vi "Set Ziro.vi"(6 "Direction":T1, 7 "init":bool, 8 "error in (no error)":errorcluster, 11 "Stand in":refnum<class "Stand.lvclass">) -> (0 "error out":errorcluster, 3 "Stand out":refnum<class "Stand.lvclass">)   [LabVIEW 2019, in "Stand.lvclass"]
uses:
  Stand.lvclass
  TypeDef/Direction.ctl
  D:/GIT H4000/H4000/src/Device_class/Device.lvclass
  Stand.lvclass/Stand.ctl
  Valve Mode.ctl
  Device_class/Device.lvclass/Device.ctl
  NeedleValve_class/Cmd.ctl
  ee99d7a0-1d06-4dde-a5e8-abf916667462.vi
  f8234472-8bf1-448c-8c25-8d9f60be58e1.vi
  6b2010b2-6e4b-4e14-9c16-a142e06b5f9e.vi
  Valve State Mode.vi
  Valve State Mode.vi/810e184e-eeb6-4027-a8ae-1422f3ce3d45.vi
  Valve State Mode.vi/57bd4a65-f3dc-44f5-8d68-677c2a197570.vi
  Valve State Mode.vi/03b2f9e4-fceb-4725-9b90-3fd10082a088.vi
  Valve State Mode.vi/2785bab5-dd59-4d13-b638-b9157202fa4a.vi
  Valve State Mode.vi/50faa4b8-a9b4-4cc6-ab66-55c42b424fcd.vi
  Valve State Mode.vi/c882c3fe-b7a7-4419-8f9b-6788aa23338b.vi
  Valve State Mode.vi/3d0d09bd-48e8-482f-b1e2-a36b2bb65234.vi
  Valve State Mode.vi/33d3f26a-dc4a-4f56-bf0a-61d04c5d7434.vi
  Valve State Mode.vi/52af9d47-24d1-4057-80bf-8d93bfb3d17d.vi
  Valve State Mode.vi/bbc9916c-129f-4456-975e-9c3ae3d5db66.vi
  Valve State Mode.vi/a6106d78-2bf9-477e-b655-d47fad07ddfe.vi
  Valve State Mode.vi/e2916439-03c6-4471-bb40-42242a636e27.vi
  Valve State Mode.vi/094228cb-a119-423c-9af8-5a16f059a318.vi
  Valve State Mode.vi/bf5ad1e6-a0ae-4579-ad74-ca8f304cb7cf.vi
  Valve State Mode.vi/eb4d2b76-f0f0-4e1d-bda0-609c5f37b4e7.vi
  Const All Valve.vi
  FPGA/TypeDef/DO index.ctl
  FPGA_API_class/FPGA API.lvclass
  Device_class/Device.lvclass
  NeedleValve_class/NeedleValve.lvclass
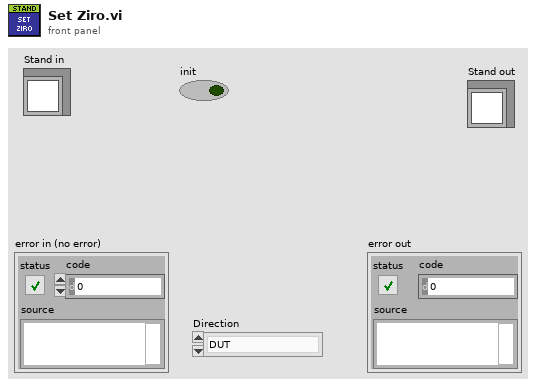
[diagram p1: front panel]
types:
  T1 = typedef "Direction.ctl" = enum8{"DUT", "Chamber"}
  T2 = typedef "DO index.ctl" = u8
  T3 = typedef "SP_TYPE.ctl" = enum16{"ERROR", "ZIRO", "BASE", "SP"}
  T4 = typedef "Valve Mode.ctl" = enum16{"Filling DUT", "Filling Chamber", "Pump Pressure DUT", "Pump Pressure Chamber", "Haskel Pressure DUT", "Haskel Pressure Chamber", "Slow Release DUT", "Slow Release Chamber", "Fast Release DUT", "Fast Release Chamber", "Fast Release DUT and Chamber", "Leak Pressure DUT", "Leak Pressure Chamber", "Back Pressure DUT", "Back Pressure Chamber", "Fully Closed", "Drain", "Block DUT", "Block Chamber", "filling dut down", "filling chamber down"}
  T5 = typedef "NeedleValve.lvclass/Cmd.ctl" = enum16{"Open", "Close", "Stop", "Prep open"}
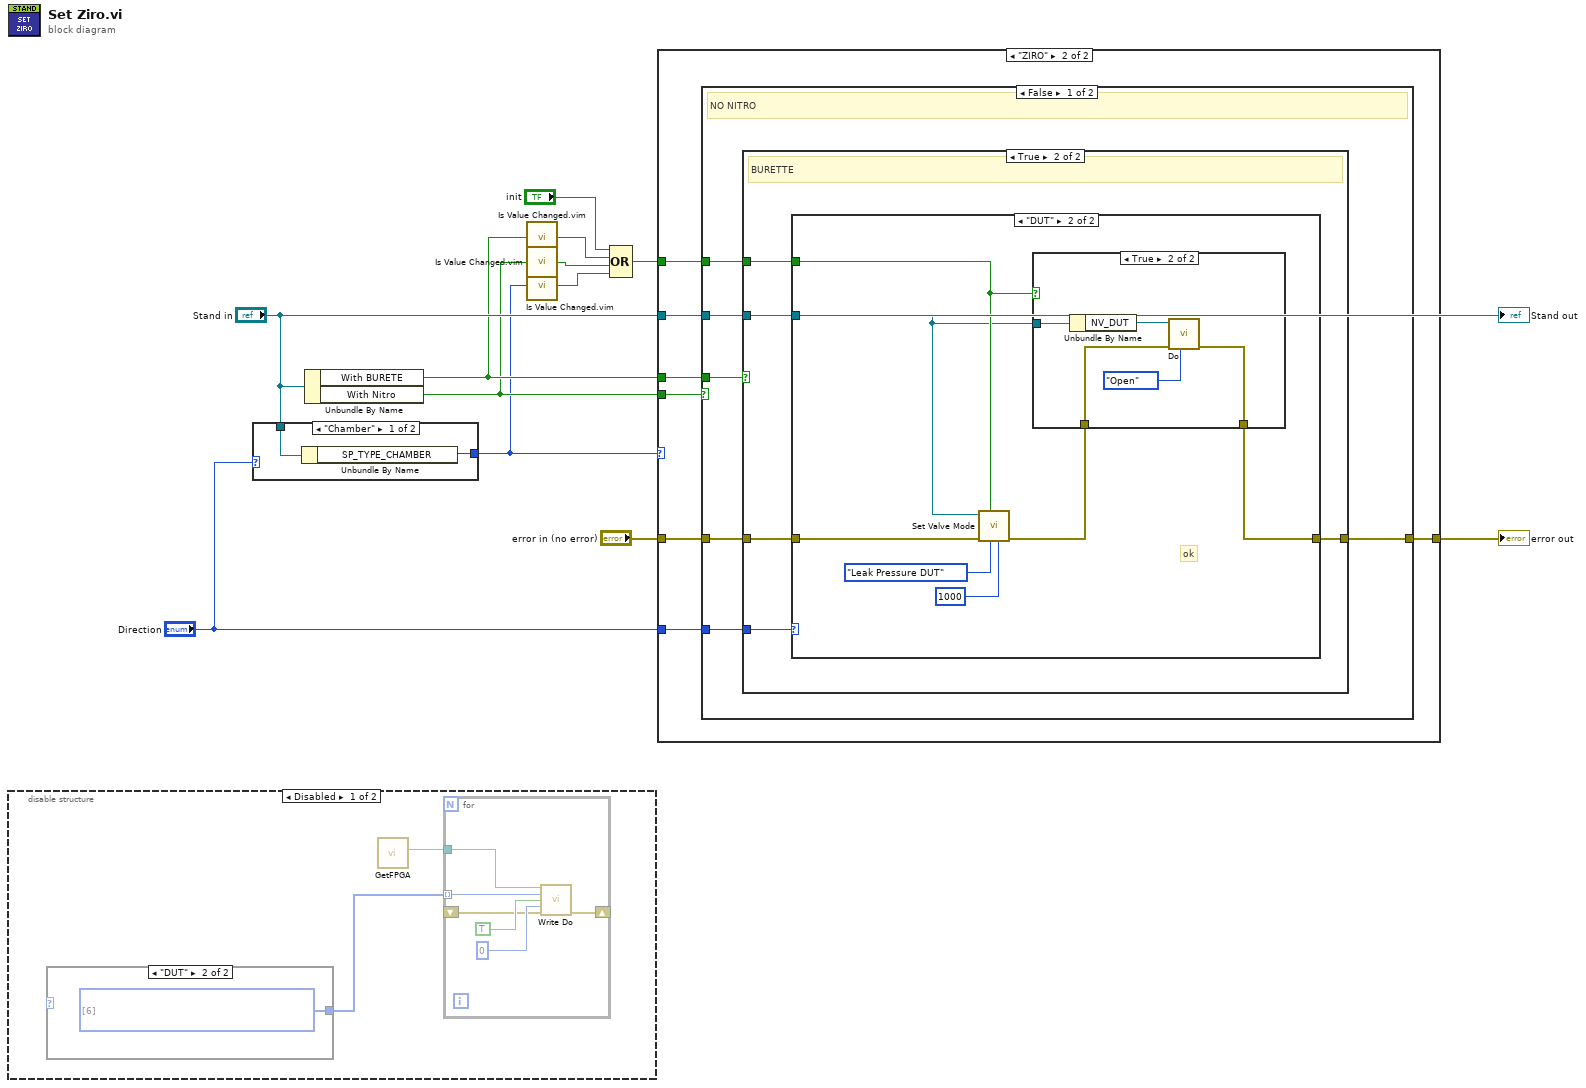
[diagram p0: block diagram]
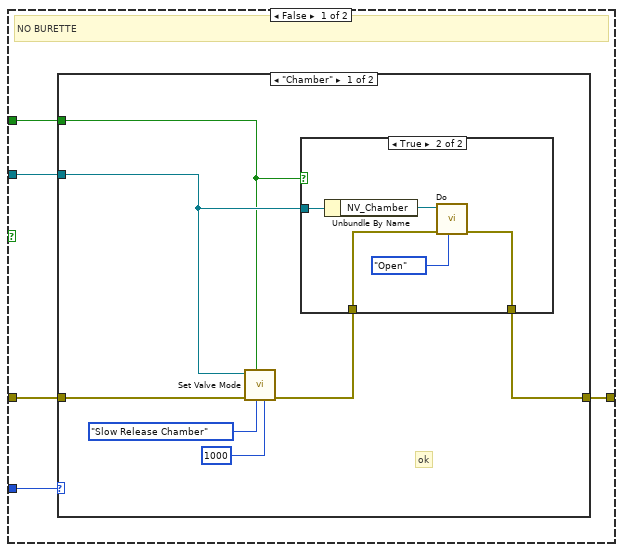
[diagram p3: hidden frame]
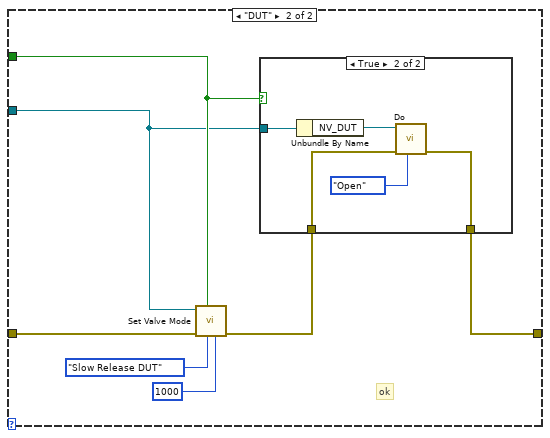
[diagram p5: hidden frame]
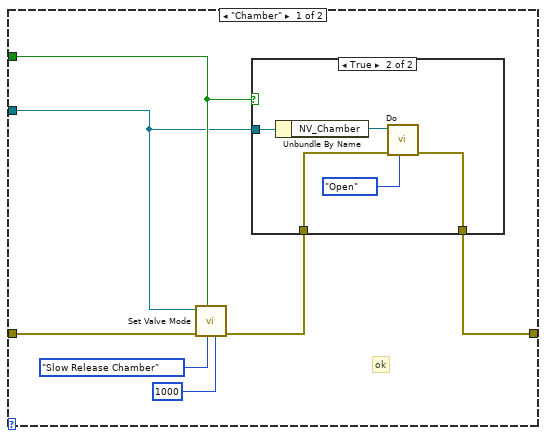
[diagram p7: hidden frame]
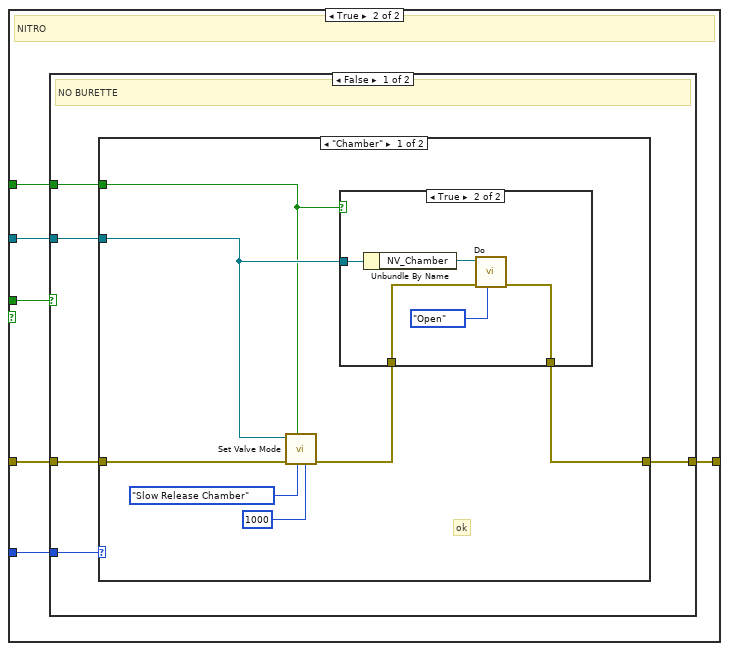
[diagram p10: hidden frame]
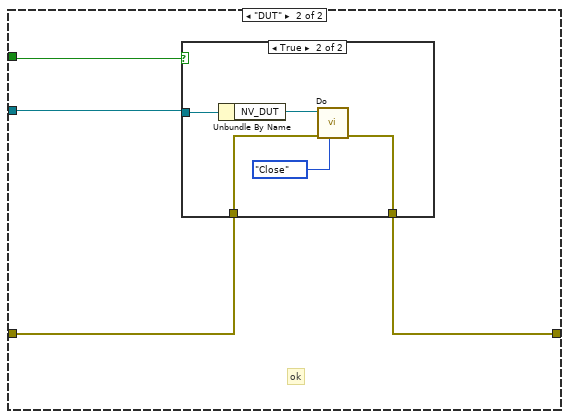
[diagram p12: hidden frame]
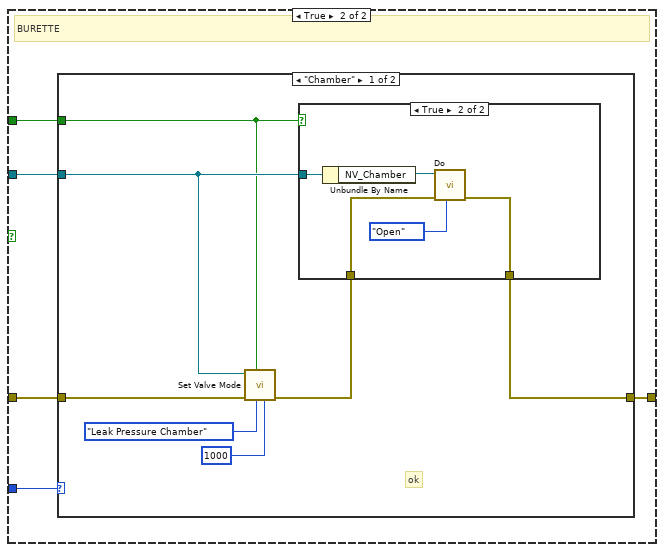
[diagram p14: hidden frame]
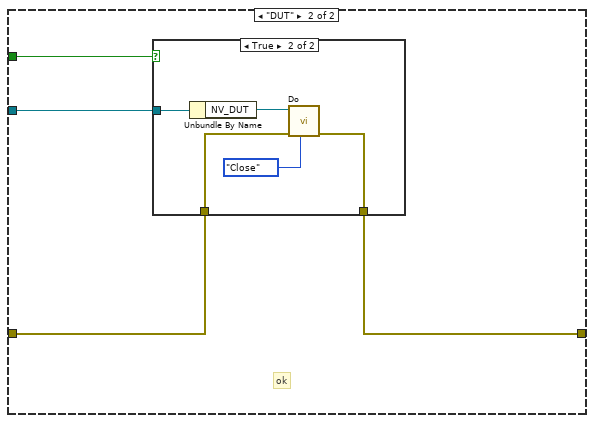
[diagram p16: hidden frame]
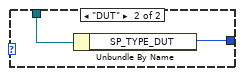
[diagram p18: hidden frame]
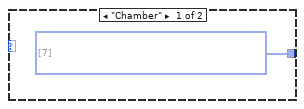
[diagram p19: hidden frame]
diagram:
  n1 = disable-structure shown="Disabled" {
    frame Disabled {
      n2 = case shown="\"DUT\"" {
        selector: _ -> [_ _]
        tunnel: [w21 w22] -> w13
        frame "Chamber" {
          w21 = T2[] [7] items=["DO 0 [KP1] [M12]", "DO 1 [ON KP2] [M21]", "DO 2 [ON KP3] [M24]", "DO 3 [WATER Y18.1 [DO3]]", "DO 4 [WATER Y18.2 [DO4]]", "DO 5 [KP6 Y29.1 33.7]", "DO 6 [KP7 Y29.2 33.8]", "DO 7 [KP8 Y29.3 33.9]", "DO 8 [KP9 Y29.4  33.12]", "DO 9 [KP10 Y29.5 33.1]", "DO 10 [KP11 Y29.6 33.2]", "DO 11 [KP12 Y29.7  33.13]", "DO 12 [KP13 Y29.8  33.11]", "DO 13 [KP14 Y29.9 33.10]", "DO 14 [KP15 Y29.10  33.6]", "DO 15 [KP16 Y29.11  33.5]", "DO 16 [KP17 Y29.12  33.4]", "DO 17 [KP18 Y29.13 33.3]", "DO 18 [AIR KP19]", "DO 19 [STEP DRIVE EN KP20]", "DO 20 [KP21 Y44.1 OPEN]", "DO 21 [ KP22 Y44.1 CLOSE]", "DO 22 [ KP23 Y44.2 OPEN]", "DO 23", "DO 24 [STEP DRIVE 1]", "DO 25 [STEP DRIVE 2]"]
        }
        frame "DUT" {
          w22 = T2[] [6] items=["DO 0 [KP1] [M12]", "DO 1 [ON KP2] [M21]", "DO 2 [ON KP3] [M24]", "DO 3 [WATER Y18.1 [DO3]]", "DO 4 [WATER Y18.2 [DO4]]", "DO 5 [KP6 Y29.1 33.7]", "DO 6 [KP7 Y29.2 33.8]", "DO 7 [KP8 Y29.3 33.9]", "DO 8 [KP9 Y29.4  33.12]", "DO 9 [KP10 Y29.5 33.1]", "DO 10 [KP11 Y29.6 33.2]", "DO 11 [KP12 Y29.7  33.13]", "DO 12 [KP13 Y29.8  33.11]", "DO 13 [KP14 Y29.9 33.10]", "DO 14 [KP15 Y29.10  33.6]", "DO 15 [KP16 Y29.11  33.5]", "DO 16 [KP17 Y29.12  33.4]", "DO 17 [KP18 Y29.13 33.3]", "DO 18 [AIR KP19]", "DO 19 [STEP DRIVE EN KP20]", "DO 20 [KP21 Y44.1 OPEN]", "DO 21 [ KP22 Y44.1 CLOSE]", "DO 22 [ KP23 Y44.2 OPEN]", "DO 23", "DO 24 [STEP DRIVE 1]", "DO 25 [STEP DRIVE 2]"]
        }
      }
      n3 = call "GetFPGA.vi"() -> ("FPGA API.lvclass"=w14:refnum<class "FPGA API.lvclass">)  [unwired: 11 in]
      n4 = for {
        tunnel: w14 -> [w18]
        tunnel: w13 -> [w16] mode=indexing
        shift-right: [w15] -> _
        shift-left: _ -> [w17]
        n5 = call-dynamic "Write Do.vi"("FPGA API in"=w18, "#DO"=w16, "value"=TRUE, "Time uSec"=u32 0, "error in (no error)"=w17) -> ("error out"=w15:errorcluster)  [unwired: 9 in, 1 out]
      }
    }
    frame Enabled {
    }
  }
  n6 = case shown="\"Chamber\"" "Direction" {
    tunnel: [w24 w26] -> w2
    tunnel: "Stand in" -> [w23 w25]
    frame "Chamber" {
      n7 = Unbundle By Name(w23) -> ("SP_TYPE_CHAMBER"=w24:T3)
    }
    frame "DUT" {
      n8 = Unbundle By Name(w25) -> ("SP_TYPE_DUT"=w26:T3)
    }
  }
  n9 = Unbundle By Name("Stand in") -> ("With BURETE"=w8:bool, "With Nitro"=w4:bool)
  n10 = call "Is Value Changed.vim"("value"=w8) -> ("changed or first call?"=w6:bool)
  n11 = call "Is Value Changed.vim"("value"=w4) -> ("changed or first call?"=w3:bool)
  n12 = call "Is Value Changed.vim"("value"=w2) -> ("changed or first call?"=w1:bool)
  n13 = Compound Arithmetic op=OR("init", w6, w3, w1) -> (w5:bool)
  n14 = case shown="\"ZIRO\"" w2 {
    tunnel: "Stand in" -> [_ w34]
    tunnel: [w27 w31] -> w11
    tunnel: "error in (no error)" -> [w27 w32]
    tunnel: "Direction" -> [_ w30]
    tunnel: w8 -> [_ w29]
    tunnel: w5 -> [_ w33]
    tunnel: w4 -> [_ w28]
    frame Default {
    }
    frame "ZIRO" {
      n15 = case shown="False" w28 {
        tunnel: w34 -> [w40 w108]
        tunnel: w33 -> [w39 w107]
        tunnel: w32 -> [w38 w106]
        tunnel: [w37 w105] -> w31
        tunnel: w30 -> [w36 w104]
        tunnel: w29 -> [w35 w103]
        frame False {
          # "NO NITRO"
          n16 = case shown="True" w35 {
            tunnel: w40 -> [w45 w76]
            tunnel: w39 -> [w44 w75]
            tunnel: w38 -> [w43 w74]
            tunnel: [w42 w73] -> w37
            tunnel: w36 -> [w41 w72]
            frame False {
              # "NO BURETTE"
              n17 = case shown="\"Chamber\"" w41 {
                tunnel: w45 -> [w49 w61]
                tunnel: w44 -> [w46 w62]
                tunnel: w43 -> [w51 w64]
                tunnel: [w47 w59] -> w42
                frame "Chamber" {
                  # "ok"
                  n18 = call "Set Valve Mode.vi"("time after close"=u32 1000, "Valve DIR"=Valve_Mode."Slow Release Chamber", "init"=w46, "error in (no error)"=w51, "Stand in"=w49) -> ("error out"=w48:errorcluster)  [unwired: 5 in, 1 out]
                  n19 = case shown="True" w46 {
                    tunnel: w49 -> [_ w58]
                    tunnel: w48 -> [w53 w57]
                    tunnel: [w53 w56] -> w47
                    frame False {
                    }
                    frame True {
                      n20 = Unbundle By Name(w58) -> ("NV_Chamber"=w55:refnum<class "NeedleValve.lvclass">)
                      n21 = call "Do.vi"("Cmd"=Cmd."Open", "error in (no error)"=w57, "NeedleValve in"=w55) -> ("error out"=w56:errorcluster)  [unwired: 7 in, 1 out]
                    }
                  }
                }
                frame "DUT" {
                  # "ok"
                  n22 = call "Set Valve Mode.vi"("time after close"=u32 1000, "Valve DIR"=Valve_Mode."Slow Release DUT", "init"=w62, "error in (no error)"=w64, "Stand in"=w61) -> ("error out"=w60:errorcluster)  [unwired: 5 in, 1 out]
                  n23 = case shown="True" w62 {
                    tunnel: w61 -> [_ w71]
                    tunnel: w60 -> [w66 w70]
                    tunnel: [w66 w69] -> w59
                    frame False {
                    }
                    frame True {
                      n24 = Unbundle By Name(w71) -> ("NV_DUT"=w68:refnum<class "NeedleValve.lvclass">)
                      n25 = call "Do.vi"("Cmd"=Cmd."Open", "error in (no error)"=w70, "NeedleValve in"=w68) -> ("error out"=w69:errorcluster)  [unwired: 7 in, 1 out]
                    }
                  }
                }
              }
            }
            frame True {
              # "BURETTE"
              n26 = case shown="\"DUT\"" w72 {
                tunnel: w76 -> [w79 w90]
                tunnel: w75 -> [w80 w93]
                tunnel: w74 -> [w82 w95]
                tunnel: [w77 w91] -> w73
                frame "Chamber" {
                  # "ok"
                  n27 = call "Set Valve Mode.vi"("time after close"=u32 1000, "Valve DIR"=Valve_Mode."Slow Release Chamber", "init"=w80, "error in (no error)"=w82, "Stand in"=w79) -> ("error out"=w78:errorcluster)  [unwired: 5 in, 1 out]
                  n28 = case shown="True" w80 {
                    tunnel: w79 -> [_ w89]
                    tunnel: w78 -> [w84 w88]
                    tunnel: [w84 w87] -> w77
                    frame False {
                    }
                    frame True {
                      n29 = Unbundle By Name(w89) -> ("NV_Chamber"=w86:refnum<class "NeedleValve.lvclass">)
                      n30 = call "Do.vi"("Cmd"=Cmd."Open", "error in (no error)"=w88, "NeedleValve in"=w86) -> ("error out"=w87:errorcluster)  [unwired: 7 in, 1 out]
                    }
                  }
                }
                frame "DUT" {
                  # "ok"
                  n31 = call "Set Valve Mode.vi"("time after close"=u32 1000, "Valve DIR"=Valve_Mode."Leak Pressure DUT", "init"=w93, "error in (no error)"=w95, "Stand in"=w90) -> ("error out"=w92:errorcluster)  [unwired: 5 in, 1 out]
                  n32 = case shown="True" w93 {
                    tunnel: w90 -> [_ w102]
                    tunnel: w92 -> [w97 w101]
                    tunnel: [w97 w100] -> w91
                    frame False {
                    }
                    frame True {
                      n33 = Unbundle By Name(w102) -> ("NV_DUT"=w99:refnum<class "NeedleValve.lvclass">)
                      n34 = call "Do.vi"("Cmd"=Cmd."Open", "error in (no error)"=w101, "NeedleValve in"=w99) -> ("error out"=w100:errorcluster)  [unwired: 7 in, 1 out]
                    }
                  }
                }
              }
            }
          }
        }
        frame True {
          # "NITRO"
          n35 = case shown="False" w103 {
            tunnel: w108 -> [w113 w141]
            tunnel: w107 -> [w112 w140]
            tunnel: w106 -> [w111 w139]
            tunnel: [w110 w138] -> w105
            tunnel: w104 -> [w109 w137]
            frame False {
              # "NO BURETTE"
              n36 = case shown="\"Chamber\"" w109 {
                tunnel: w113 -> [w117 w130]
                tunnel: w112 -> [w114 w129]
                tunnel: w111 -> [w119 w128]
                tunnel: [w115 w127] -> w110
                frame "Chamber" {
                  # "ok"
                  n37 = call "Set Valve Mode.vi"("time after close"=u32 1000, "Valve DIR"=Valve_Mode."Slow Release Chamber", "init"=w114, "error in (no error)"=w119, "Stand in"=w117) -> ("error out"=w116:errorcluster)  [unwired: 5 in, 1 out]
                  n38 = case shown="True" w114 {
                    tunnel: w117 -> [_ w126]
                    tunnel: w116 -> [w121 w125]
                    tunnel: [w121 w124] -> w115
                    frame False {
                    }
                    frame True {
                      n39 = Unbundle By Name(w126) -> ("NV_Chamber"=w123:refnum<class "NeedleValve.lvclass">)
                      n40 = call "Do.vi"("Cmd"=Cmd."Open", "error in (no error)"=w125, "NeedleValve in"=w123) -> ("error out"=w124:errorcluster)  [unwired: 7 in, 1 out]
                    }
                  }
                }
                frame "DUT" {
                  # "ok"
                  n41 = case shown="True" w129 {
                    tunnel: w130 -> [_ w136]
                    tunnel: w128 -> [w131 w135]
                    tunnel: [w131 w134] -> w127
                    frame False {
                    }
                    frame True {
                      n42 = Unbundle By Name(w136) -> ("NV_DUT"=w133:refnum<class "NeedleValve.lvclass">)
                      n43 = call "Do.vi"("Cmd"=Cmd."Close", "error in (no error)"=w135, "NeedleValve in"=w133) -> ("error out"=w134:errorcluster)  [unwired: 7 in, 1 out]
                    }
                  }
                }
              }
            }
            frame True {
              # "BURETTE"
              n44 = case shown="\"Chamber\"" w137 {
                tunnel: w141 -> [w145 w158]
                tunnel: w140 -> [w144 w157]
                tunnel: w139 -> [w147 w156]
                tunnel: [w142 w155] -> w138
                frame "Chamber" {
                  # "ok"
                  n45 = call "Set Valve Mode.vi"("time after close"=u32 1000, "Valve DIR"=Valve_Mode."Leak Pressure Chamber", "init"=w144, "error in (no error)"=w147, "Stand in"=w145) -> ("error out"=w143:errorcluster)  [unwired: 5 in, 1 out]
                  n46 = case shown="True" w144 {
                    tunnel: w145 -> [_ w154]
                    tunnel: w143 -> [w149 w153]
                    tunnel: [w149 w152] -> w142
                    frame False {
                    }
                    frame True {
                      n47 = Unbundle By Name(w154) -> ("NV_Chamber"=w151:refnum<class "NeedleValve.lvclass">)
                      n48 = call "Do.vi"("Cmd"=Cmd."Open", "error in (no error)"=w153, "NeedleValve in"=w151) -> ("error out"=w152:errorcluster)  [unwired: 7 in, 1 out]
                    }
                  }
                }
                frame "DUT" {
                  # "ok"
                  n49 = case shown="True" w157 {
                    tunnel: w158 -> [_ w164]
                    tunnel: w156 -> [w159 w163]
                    tunnel: [w159 w162] -> w155
                    frame False {
                    }
                    frame True {
                      n50 = Unbundle By Name(w164) -> ("NV_DUT"=w161:refnum<class "NeedleValve.lvclass">)
                      n51 = call "Do.vi"("Cmd"=Cmd."Close", "error in (no error)"=w163, "NeedleValve in"=w161) -> ("error out"=w162:errorcluster)  [unwired: 7 in, 1 out]
                    }
                  }
                }
              }
            }
          }
        }
      }
    }
  }
  "error out" <- w11
  "Stand out" <- "Stand in"
